vi "Cryomagnetics Read Field.vi"(8 "error in (no error)":errorcluster, 11 "VISA resource name":refnum<visa-resource-name>) -> (0 "error out":errorcluster, 1 "data string out":string, 2 "Field":dbl, 3 "VISA Resource Name Out":refnum<visa-resource-name>)   [LabVIEW 2015]
uses:
  GPIB/VISA  Send Receive.vi
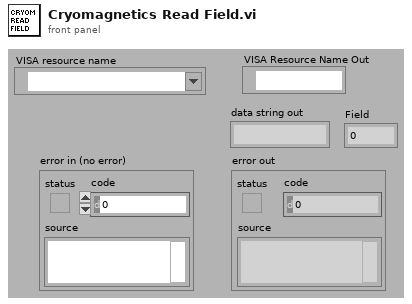
[diagram p1: front panel]
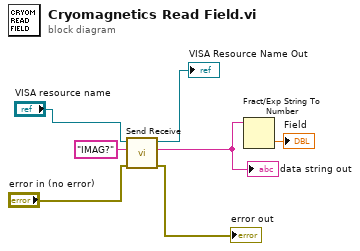
[diagram p0: block diagram]
diagram:
  n1 = call-poly "Send Receive.vi"("error in (no error)"="error in (no error)", "data string in"="IMAG?", "VISA Resource Name"="VISA resource name") -> ("error out"=→"error out":errorcluster, "data string out"=w5:string, "VISA Resource Name Out"=→"VISA Resource Name Out":refnum<visa-resource-name>)  [unwired: 6 in]
  "data string out" <- w5
  n2 = Fract/Exp String To Number(string=w5) -> (number=→"Field":dbl)  [unwired: 4 out]
